vi "Device.GetPublicEvents.vi"(8 "error in (no error)":errorcluster, 11 "Device in":refnum<class "Device.lvclass">) -> (0 "error out":errorcluster, 2 "Public Events":T1, 3 "Device out":refnum<class "Device.lvclass">)   [LabVIEW 2019, in "Device.lvclass"]
uses:
  Device.lvclass
  Typedefs/PublicEvents--Cluster.ctl
  Typedefs/PublicEvents--Device.Initialized.ctl
  Typedefs/PublicEvents--Device.Uninitialized.ctl
  Device.lvclass/Device.ctl
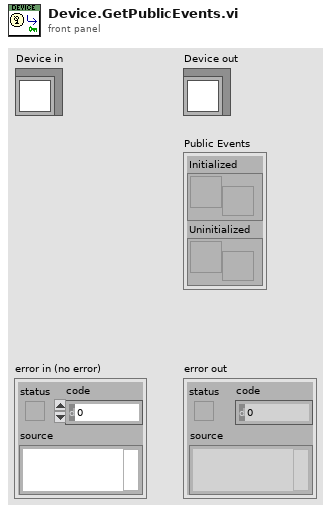
[diagram p1: front panel]
types:
  T1 = typedef "Device.lvclass/PublicEvents--Cluster.ctl" = cluster{"Initialized":refnum<user-event>, "Uninitialized":refnum<user-event>}
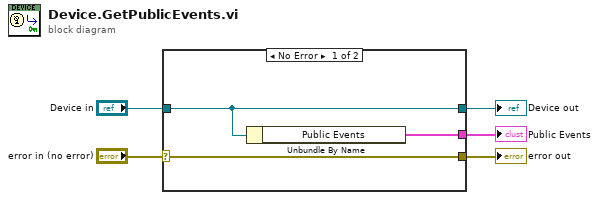
[diagram p0: block diagram]
diagram:
  n1 = case shown="No Error" "error in (no error)" {
    selector: "error in (no error)" -> [w8 w10]
    tunnel: [w8 w10] -> w4
    tunnel: [w7 w9] -> w2
    tunnel: "Device in" -> [w7 w9]
    tunnel: [w6 _] -> w1
    frame No Error {
      n2 = Unbundle By Name(w7) -> ("Public Events"=w6:T1)
    }
    frame Error {
    }
  }
  "error out" <- w4
  "Device out" <- w2
  "Public Events" <- w1
